vi "OP500_Scan Array_P.vi"(11 "Array":dbl[](array[numeric])) -> (3 "Indice du premier valeur du courant DCIR":i32)   [LabVIEW 2020]
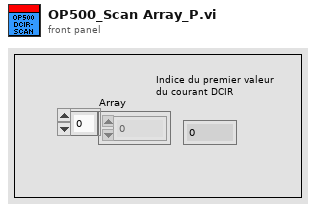
[diagram p1: front panel]
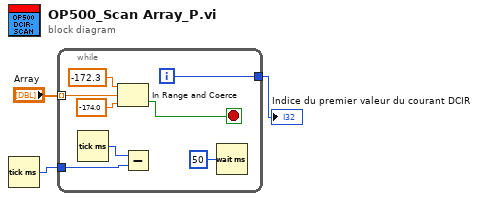
[diagram p0: block diagram]
diagram:
  n1 = Tick Count (ms)() -> (millisecond timer value=w1:u32)
  n2 = while {
    tunnel: "Array" -> [w10] mode=indexing
    tunnel: [w9] -> w3
    tunnel: w1 -> [w4]
    i -> [w9]
    stop <- w8 stop-if-true
    n3 = Tick Count (ms)() -> (millisecond timer value=w5:u32)
    n4 = In Range and Coerce(upper limit=-172.3, x=w10, lower limit=-174.0) -> (In Range?=w8:bool)  [unwired: 1 out]
    n5 = Subtract(x=w5, y=w4) -> ()  [unwired: 1 out]
    n6 = Wait (ms)(milliseconds to wait=u32 50) -> ()  [unwired: 1 out]
  }
  "Indice du premier valeur du courant DCIR" <- w3
